vi "Parse MISSION_REQUEST.vi"(11 "Data":string) -> (3 "Waypoint Number":u16)   [LabVIEW 2014]
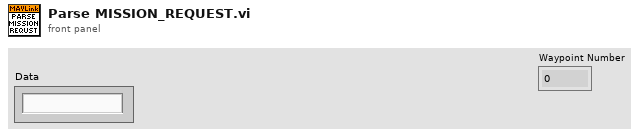
[diagram p1: front panel]
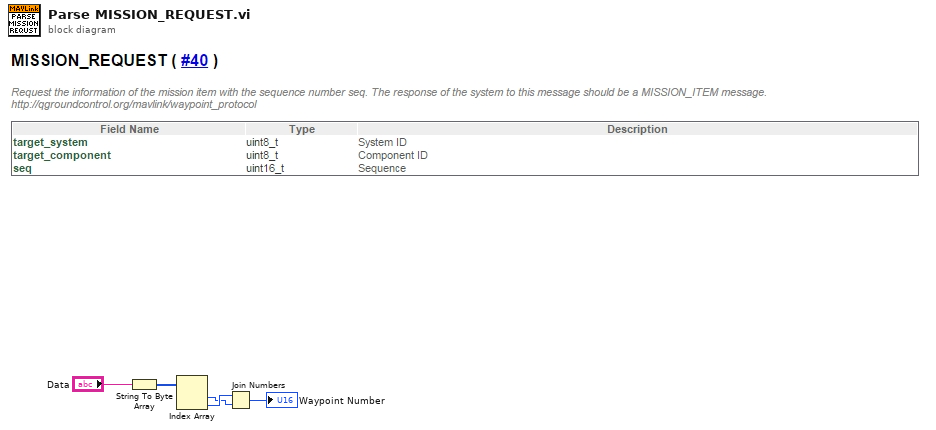
[diagram p0: block diagram]
diagram:
  n1 = String To Byte Array(string="Data") -> (unsigned byte array=w5:u8[])
  n2 = Index Array(array=w5) -> (element #1=w2:u8, element #2=w3:u8)  [unwired: 2 in]
  n3 = Join Numbers(hi=w3, lo=w2) -> ((hi.lo)=→"Waypoint Number":u16)
